vi "KeyFocus.vi"(8 "error in (no error)":errorcluster, 10 "true":bool, 11 "Array in":refnum<vi>) -> (3 "Value":variant)   [LabVIEW 2013, in "FixedChannelTBModuleDecideFeatures.lvclass"]
uses:
  FixedChannelTBModuleDecideFeatures.lvclass
panel:
  out "Label.Text":string
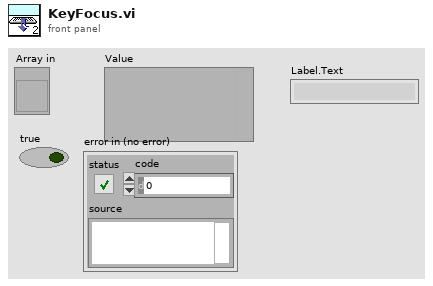
[diagram p1: front panel]
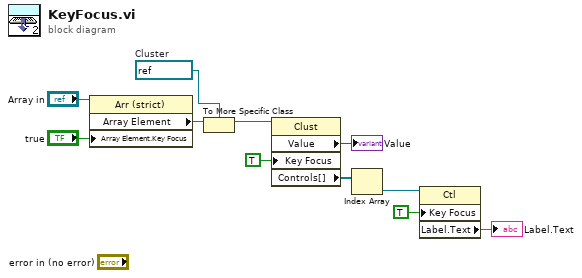
[diagram p0: block diagram]
diagram:
  w11 = refnum<vi> refnum  # Cluster
  n1 = property class="Arr (strict)"(reference="Array in", "Array Element.Key Focus"="true") -> ("Array Element"=w9:refnum<vi>)  [unwired: 1 in, 2 out]
  n2 = To More Specific Class(target class=w11, reference=w9) -> (specific class reference=w10:refnum<vi>)  [unwired: 1 in, 1 out]
  n3 = property class="Clust"(reference=w10, "Key Focus"=TRUE) -> ("Value"=→"Value":variant, "Controls[]"=w4:refnum<vi>[])  [unwired: 1 in, 2 out]
  n4 = Index Array(array=w4) -> (element=w3:refnum<vi>)  [unwired: 1 in]
  n5 = property class="Ctl"(reference=w3, "Key Focus"=TRUE) -> ("Label.Text"=→"Label.Text":string)  [unwired: 1 in, 2 out]
